vi "_Build Lens Parameters.vi"(8 "error in":errorcluster, 11 "Lens":T2[](array[typedef])) -> (0 "error out":errorcluster, 3 "Array":T1[](array[typedef]))   [LabVIEW 2015]
uses:
  Type/_XML Lens.ctl
  Type/_RT Active Ch.ctl
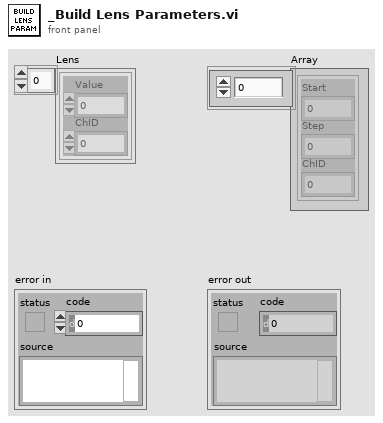
[diagram p1: front panel]
types:
  T1 = typedef "_RT Active Ch.ctl" = cluster{"Start":i32, "Step":i32, "ChID":i32}
  T2 = typedef "_XML Lens.ctl" = cluster{"Value":dbl, "ChID":u8}
  T3 = typedef "_RT Configuration 2.ctl" = cluster{"Name":string, "Ch#":u8, "Min":dbl, "Max":dbl, "Def+":dbl, "Def-":dbl, "Offset":dbl, "Slope":dbl, "Type":u8, "Description":string, "SettleT":dbl}
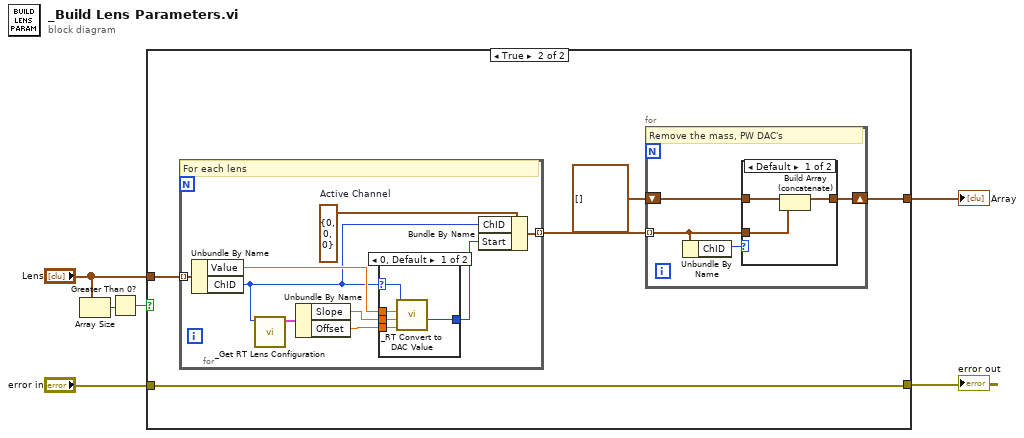
[diagram p0: block diagram]
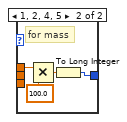
[diagram p4: hidden frame]
diagram:
  n1 = Array Size(array="Lens") -> (size(s)=w5:i32)
  n2 = Greater Than 0?(x=w5) -> (x > 0?=w4:bool)
  n3 = case shown="True" w4 {
    tunnel: "Lens" -> [_ w11]
    tunnel: "error in" -> [w7 w10]
    tunnel: [w7 w10] -> w2
    tunnel: [_ w8] -> w1
    frame False {
    }
    frame True {
      n4 = for {
        tunnel: [w25] -> w12 mode=indexing
        tunnel: w11 -> [w24] mode=indexing
        w27 = T1 {"Start"=0, "Step"=0, "ChID"=0}  # Active Channel
        # "For each lens"
        n5 = Unbundle By Name(w24) -> ("Value"=w23:dbl, "ChID"=w22:u8)
        n6 = call "_Get RT Lens Configuration.vi"("Channel #"=w22) -> ("Lens Configuration"=w21:T3)  [unwired: 5 in, 1 out]
        n7 = Unbundle By Name(w21) -> ("Slope"=w29:dbl, "Offset"=w28:dbl)
        n8 = case shown="0, Default" w22 {
          selector: w22 -> [w30 _]
          tunnel: w23 -> [w34 w38]
          tunnel: w29 -> [w33 _]
          tunnel: w28 -> [w32 _]
          tunnel: [w31 w35] -> w26
          frame 0, Default {
            n9 = call "_RT Convert to DAC Value.vi"("Offset"=w32, "Slop"=w33, "Number"=w34, "Channel"=w30) -> ("DAC Value"=w31:i32)  [unwired: 2 in, 5 out]
          }
          frame 1, 2, 4, 5 {
            # "for mass"
            n10 = Multiply(x=w38, y=100.0) -> (x*y=w36:dbl)
            n11 = To Long Integer(number=w36) -> (32bit integer=w35:i32)
          }
        }
        n12 = Bundle By Name(cluster=w27, "ChID"=w22, "Start"=w26) -> (w25:T1)
      }
      n13 = for {
        shift-right: [w14] -> w8
        shift-left: T1[] [] ("Array") -> [w15]
        tunnel: w12 -> [w13] mode=indexing
        # "Remove the mass, PW DAC's"
        n14 = Unbundle By Name(w13) -> ("ChID"=w16:i32)
        n15 = case shown="Default" w16 {
          tunnel: [w17 w20] -> w14
          tunnel: w15 -> [w19 w20]
          tunnel: w13 -> [w18 _]
          frame Default {
            n16 = Build Array (concatenate)(w19, w18) -> (w17:T1[])
          }
          frame 0..2, 4, 5, 7, 9 {
          }
        }
      }
    }
  }
  "error out" <- w2
  "Array" <- w1
